vi "meth.CheckRecurseLevel.vi"(0 "class.GLue in":refnum<class "class.GLue.lvclass">, 11 "error in (no error)":errorcluster) -> (4 "class.GLue out":refnum<class "class.GLue.lvclass">, 13 "Level":i32, 15 "error out":errorcluster)   [LabVIEW 2014, in "GLue.lvlib" / "class.GLue.lvclass"]
uses:
  class.GLue.lvclass
  class.GLue.lvclass/class.GLue.ctl
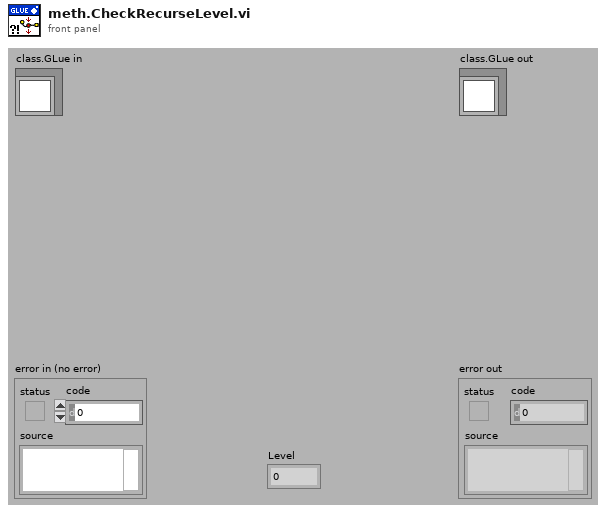
[diagram p1: front panel]
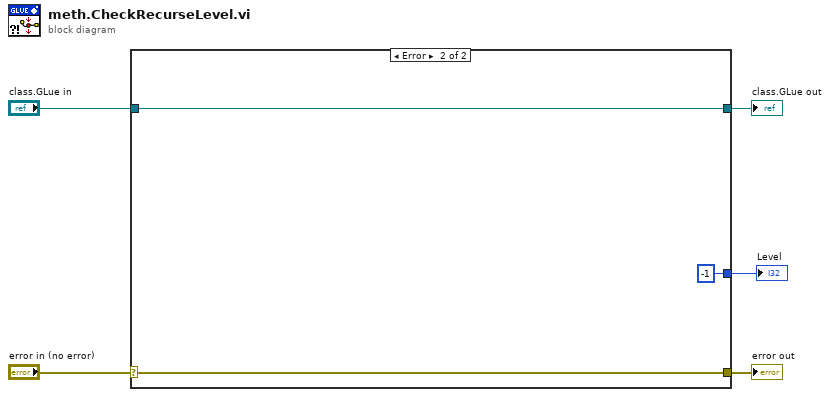
[diagram p0: block diagram]
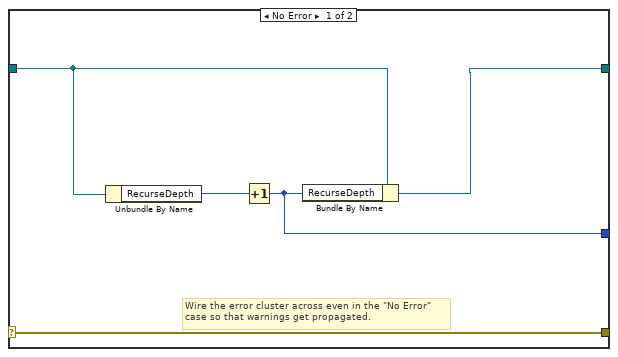
[diagram p2: hidden frame]
diagram:
  n1 = case shown="Error" "error in (no error)" {
    selector: "error in (no error)" -> [w10 w13]
    tunnel: [w10 w13] -> w4
    tunnel: [w7 w12] -> w2
    tunnel: "class.GLue in" -> [w8 w12]
    tunnel: [w6 -1] -> w1
    frame No Error {
      # "Wire the error cluster across even in the \"No Error\"\ncase so that warnings get propagated."
      n2 = Unbundle By Name(w8) -> ("RecurseDepth"=w9:i32)
      n3 = Increment(x=w9) -> (x+1=w6:i32)
      n4 = Bundle By Name(cluster=w8, "RecurseDepth"=w6) -> (w7:refnum<class "class.GLue.lvclass">)
    }
    frame Error {
    }
  }
  "error out" <- w4
  "class.GLue out" <- w2
  "Level" <- w1
